vi "Stepper_Alternative.vi"() -> ()   [LabVIEW 2013]
uses:
  <vilib>/LabVIEW Interface for Arduino/LabVIEW Interface for Arduino.lvlib
panel:
  out "Pin Values":bool[](array[boolean])
  in  "Digital I/O Pin 5":u8=7
  in  "Digital I/O Pin 4":u8=6
  in  "Digital I/O Pin 3":u8=5
  in  "Digital I/O Pin 2":u8=4
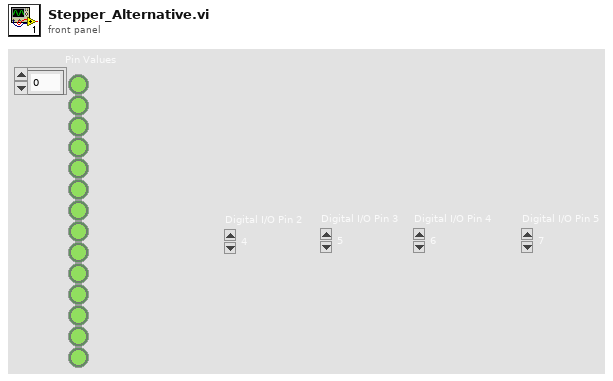
[diagram p1: front panel]
types:
  T1 = typedef "LabVIEW Interface for Arduino.lvlib/Arduino Resource.ctl" = cluster{"VISA resource":refnum<visa-resource-name>, "Board Type":T2, "Connection Type":enum8{"USB / Serial"}, "Bytes Per Packet (15)":u8}
  T2 = typedef "LabVIEW Interface for Arduino.lvlib/Board Type.ctl" = enum16{"Uno", "Dimuelanove w/Atmega 328", "Mega 2560"}
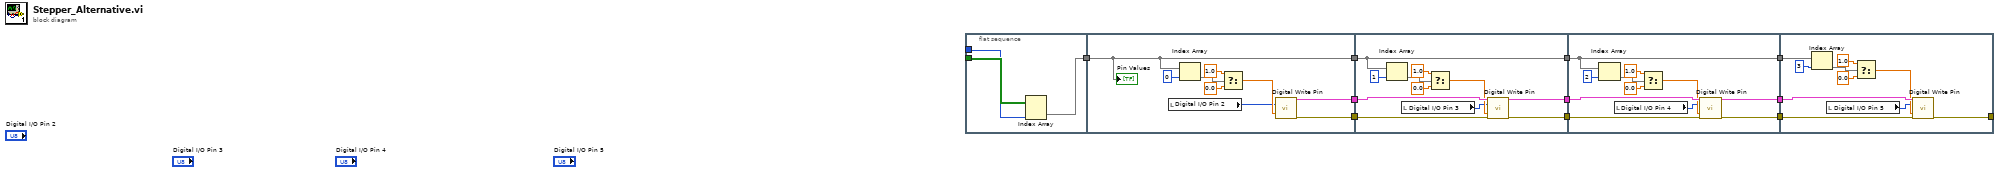
[diagram p0: block diagram]
diagram:
  n1 = flat-sequence {
    tunnel: _ -> [w13]
    tunnel: _ -> [w11]
    tunnel: [w12] -> w10
    tunnel: [w22] -> w9
    tunnel: [w21] -> w8
    tunnel: [w14] -> w7
    tunnel: w10 -> [w14]
    tunnel: w9 -> [w33]
    tunnel: [w32] -> w6
    tunnel: w8 -> [w31]
    tunnel: [w30] -> w5
    tunnel: w7 -> [w23]
    tunnel: [w23] -> w4
    tunnel: w6 -> [w44]
    tunnel: [w43] -> w3
    tunnel: w5 -> [w42]
    tunnel: [w41] -> w2
    tunnel: w4 -> [w34]
    tunnel: [w34] -> w1
    tunnel: w3 -> [w54]
    tunnel: w2 -> [w53]
    tunnel: [w52] -> _
    tunnel: w1 -> [w45]
    frame #0 {
      n2 = Index Array(array=w13, index (col)=w11) -> (element=w12)  [unwired: 1 in]
    }
    frame #1 {
      n3 = local read "Digital I/O Pin 2"() -> (w15:u8)
      n4 = Index Array(array=w14, index=0) -> (element=w20)
      n5 = Select(t=1.0, s=w20, f=0.0) -> (s? t:f=w17:dbl)
      n6 = call <vilib>:"Digital Write Pin.vi"("Digital I/O Pin (0)"=w15, "Value (0)"=w17) -> ("Arduino Resource"=w22:T1, "error out"=w21:errorcluster)  [unwired: 12 in]
      "Pin Values" <- w14
    }
    frame #2 {
      n7 = Index Array(array=w23, index=1) -> (element=w26)
      n8 = local read "Digital I/O Pin 3"() -> (w24:u8)
      n9 = Select(t=1.0, s=w26, f=0.0) -> (s? t:f=w25:dbl)
      n10 = call <vilib>:"Digital Write Pin.vi"("Arduino Resource"=w33, "Digital I/O Pin (0)"=w24, "Value (0)"=w25, "error in"=w31) -> ("Arduino Resource"=w32:T1, "error out"=w30:errorcluster)  [unwired: 10 in]
    }
    frame #3 {
      n11 = Index Array(array=w34, index=2) -> (element=w40)
      n12 = local read "Digital I/O Pin 4"() -> (w35:u8)
      n13 = Select(t=1.0, s=w40, f=0.0) -> (s? t:f=w36:dbl)
      n14 = call <vilib>:"Digital Write Pin.vi"("Arduino Resource"=w44, "Digital I/O Pin (0)"=w35, "Value (0)"=w36, "error in"=w42) -> ("Arduino Resource"=w43:T1, "error out"=w41:errorcluster)  [unwired: 10 in]
    }
    frame #4 {
      n15 = Index Array(array=w45, index=3) -> (element=w48)
      n16 = local read "Digital I/O Pin 5"() -> (w46:u8)
      n17 = Select(t=1.0, s=w48, f=0.0) -> (s? t:f=w47:dbl)
      n18 = call <vilib>:"Digital Write Pin.vi"("Arduino Resource"=w54, "Digital I/O Pin (0)"=w46, "Value (0)"=w47, "error in"=w53) -> ("error out"=w52:errorcluster)  [unwired: 10 in, 1 out]
    }
  }
